vi "MSTAutoSummary.vi"() -> ()   [LabVIEW 2012]
uses:
  <vilib>/Utility/NIReport.llb/NI_report.lvclass
  <vilib>/addons/database/Connection.llb/DB Tools Open Connec (Path).vi
  <vilib>/addons/database/Connection.llb/Conn Execute.vi
  <vilib>/addons/database/Recordset.llb/Rec Fetch Recordset Data (R).vi
  <vilib>/addons/database/Recordset.llb/Rec Destroy - Connection.vi
  <vilib>/Utility/NIReport.llb/Append Text Table to Report (wrap).vi
  <vilib>/addons/database/_DB Variant To Data/Database Variant To Data.xnode
  <vilib>/addons/database/NI_Database_API.lvlib
  <vilib>/Utility/NIReport.llb/Excel/NI_Excel.lvclass
  <vilib>/addons/_office/NI_ReportGenerationToolkit.lvlib
  <vilib>/Utility/SMTP/NI_SMTPEmail.lvlib
panel:
  in  "Report Template":path=path "O:/Monitor/Report/MSTDailyReport.xls"
  in  "Table Control":string[][](table)
  in  "Table Control 2":string[][](table)
  in  "Table Control 3":string[][](table)
  out "error out 4":errorcluster
  out "error out 5":errorcluster
  out "appended array 4":string[](array[string])
  out "recordset data 4":variant[][](array[variant])
  out "error out 3":errorcluster
  out "appended array 3":string[](array[string])
  out "recordset data 3":variant[][](array[variant])
  out "error out":errorcluster
  out "appended array":string[](array[string])
  out "recordset data":variant[][](array[variant])
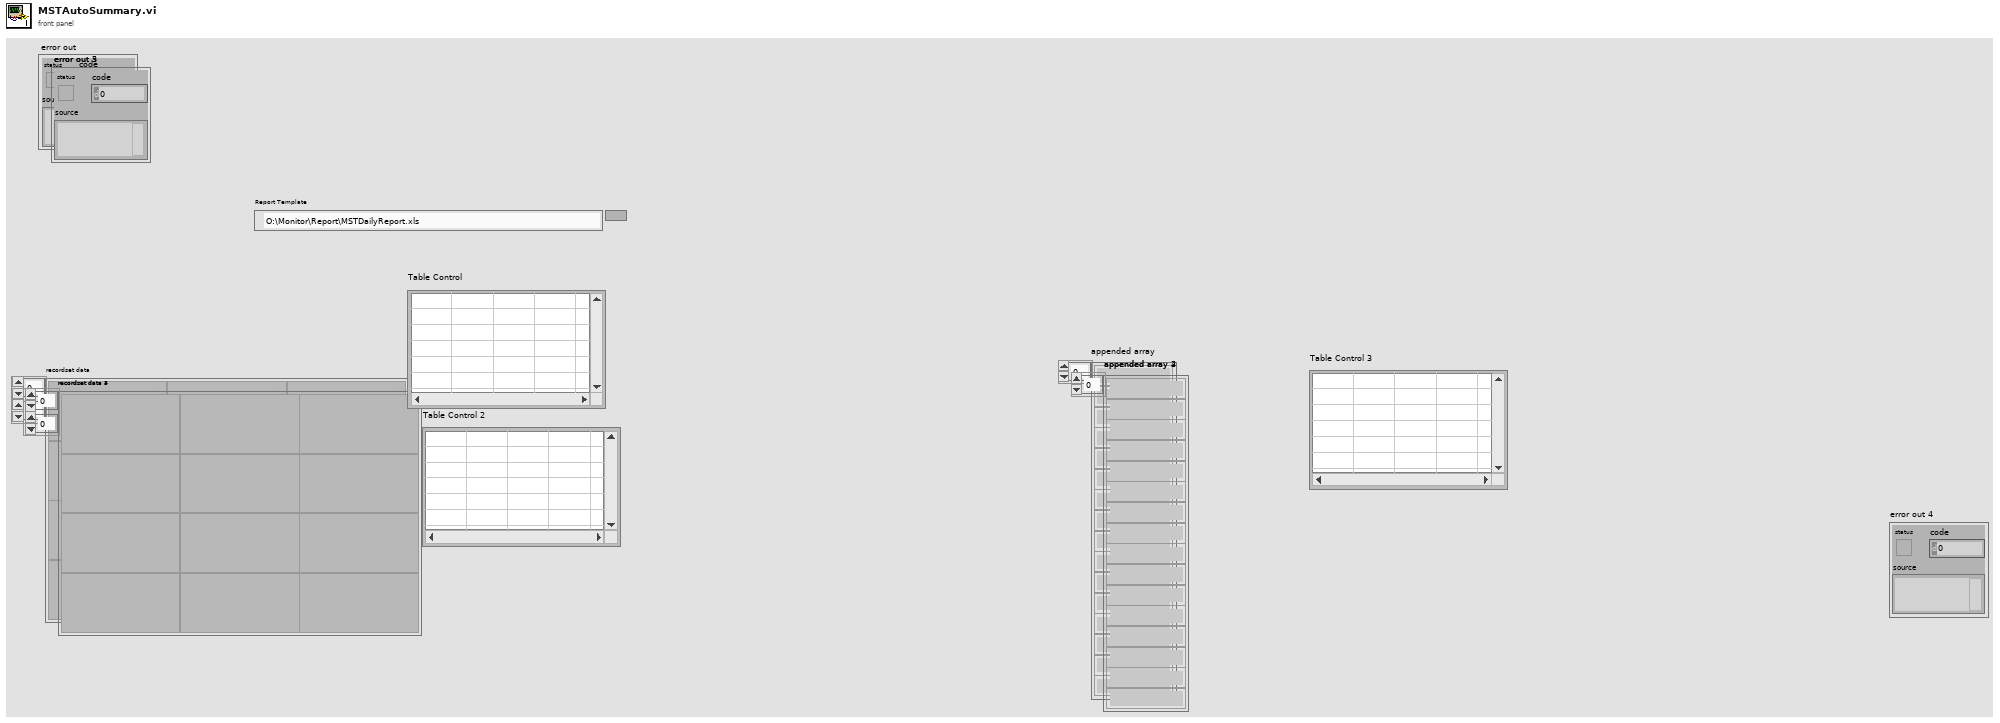
[diagram p1: front panel]
types:
  T1 = typedef "NI_Database_API.lvlib/Conn ObjectReference.ctl" = refnum<k1>
  T2 = typedef "NI_Database_API.lvlib/Rec ObjectReference.ctl" = refnum<k1>
  T3 = enum16{"Standard Report", "HTML", "Word", "Excel"}
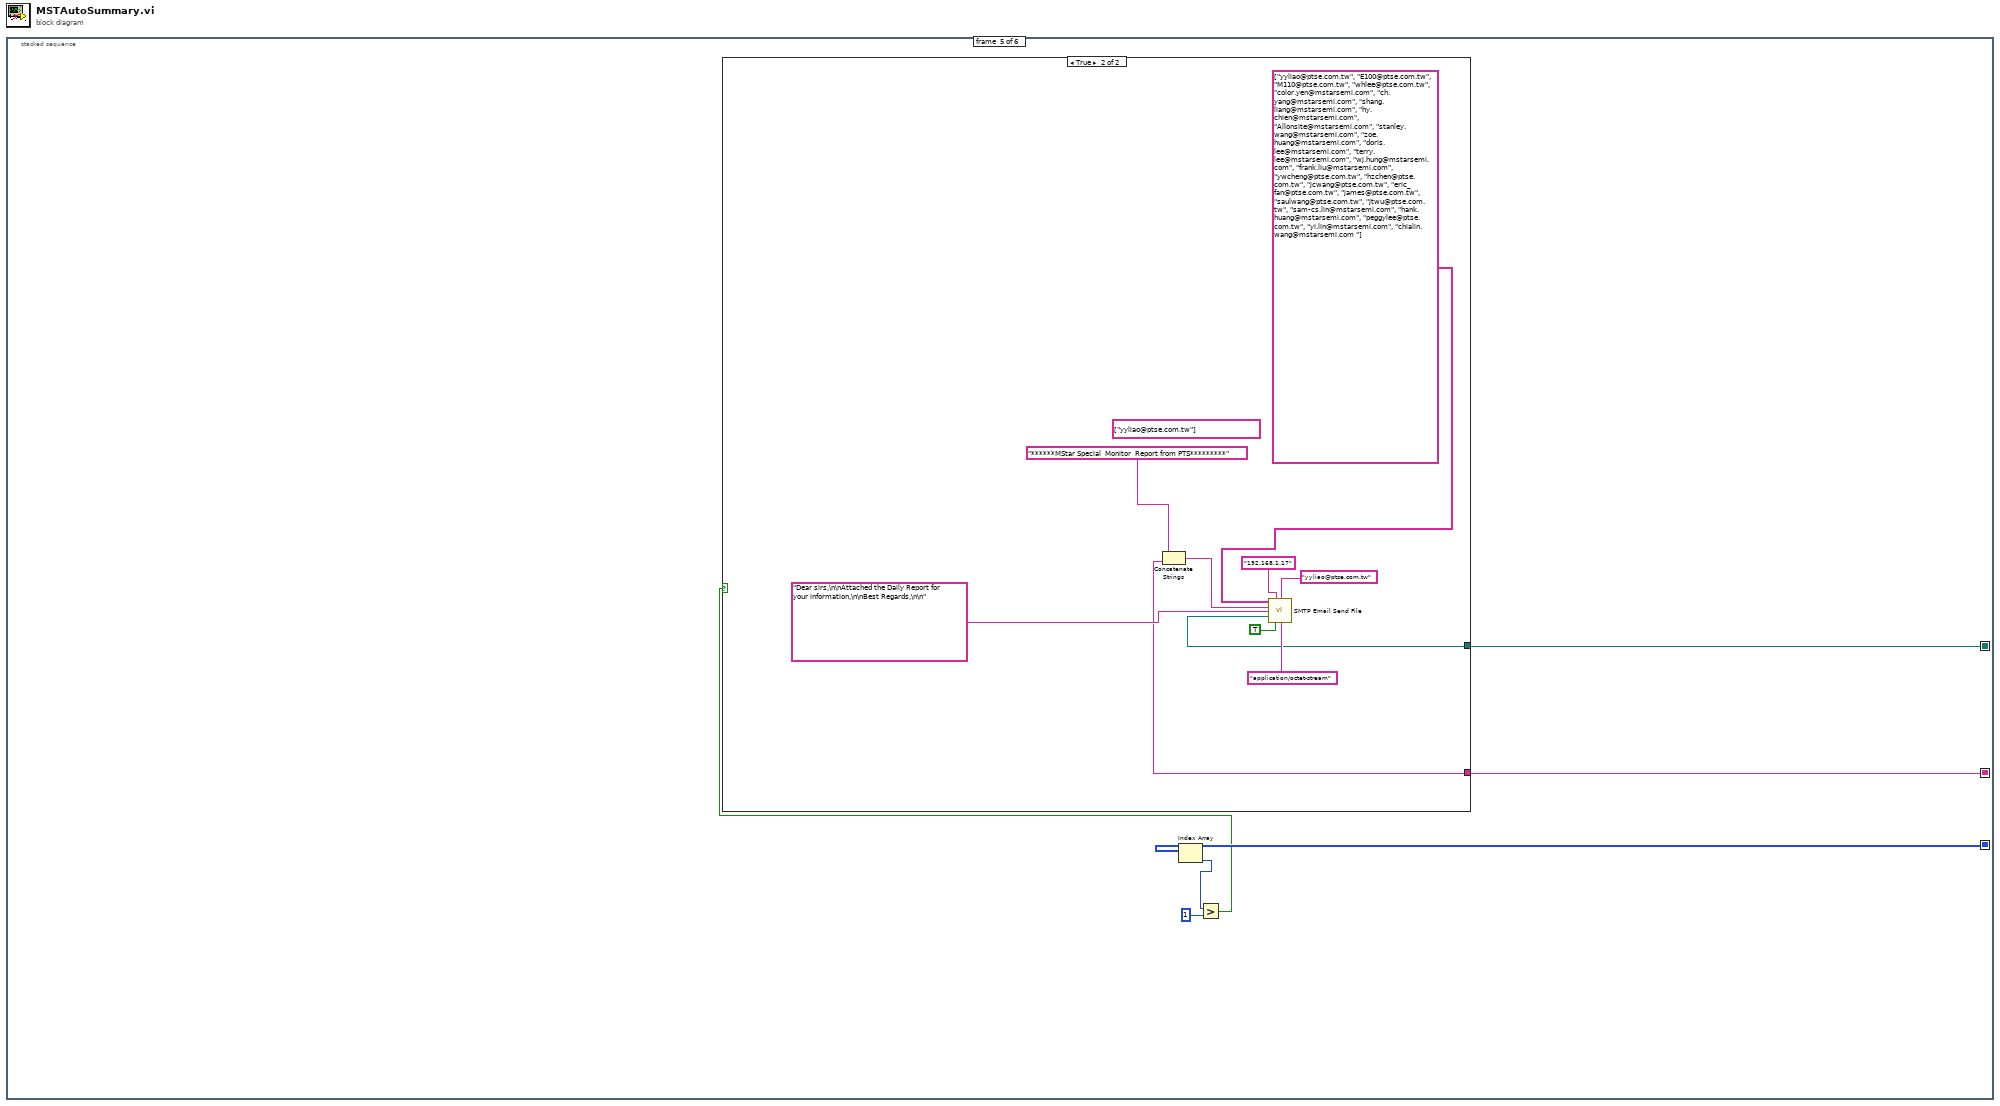
[diagram p0: block diagram]
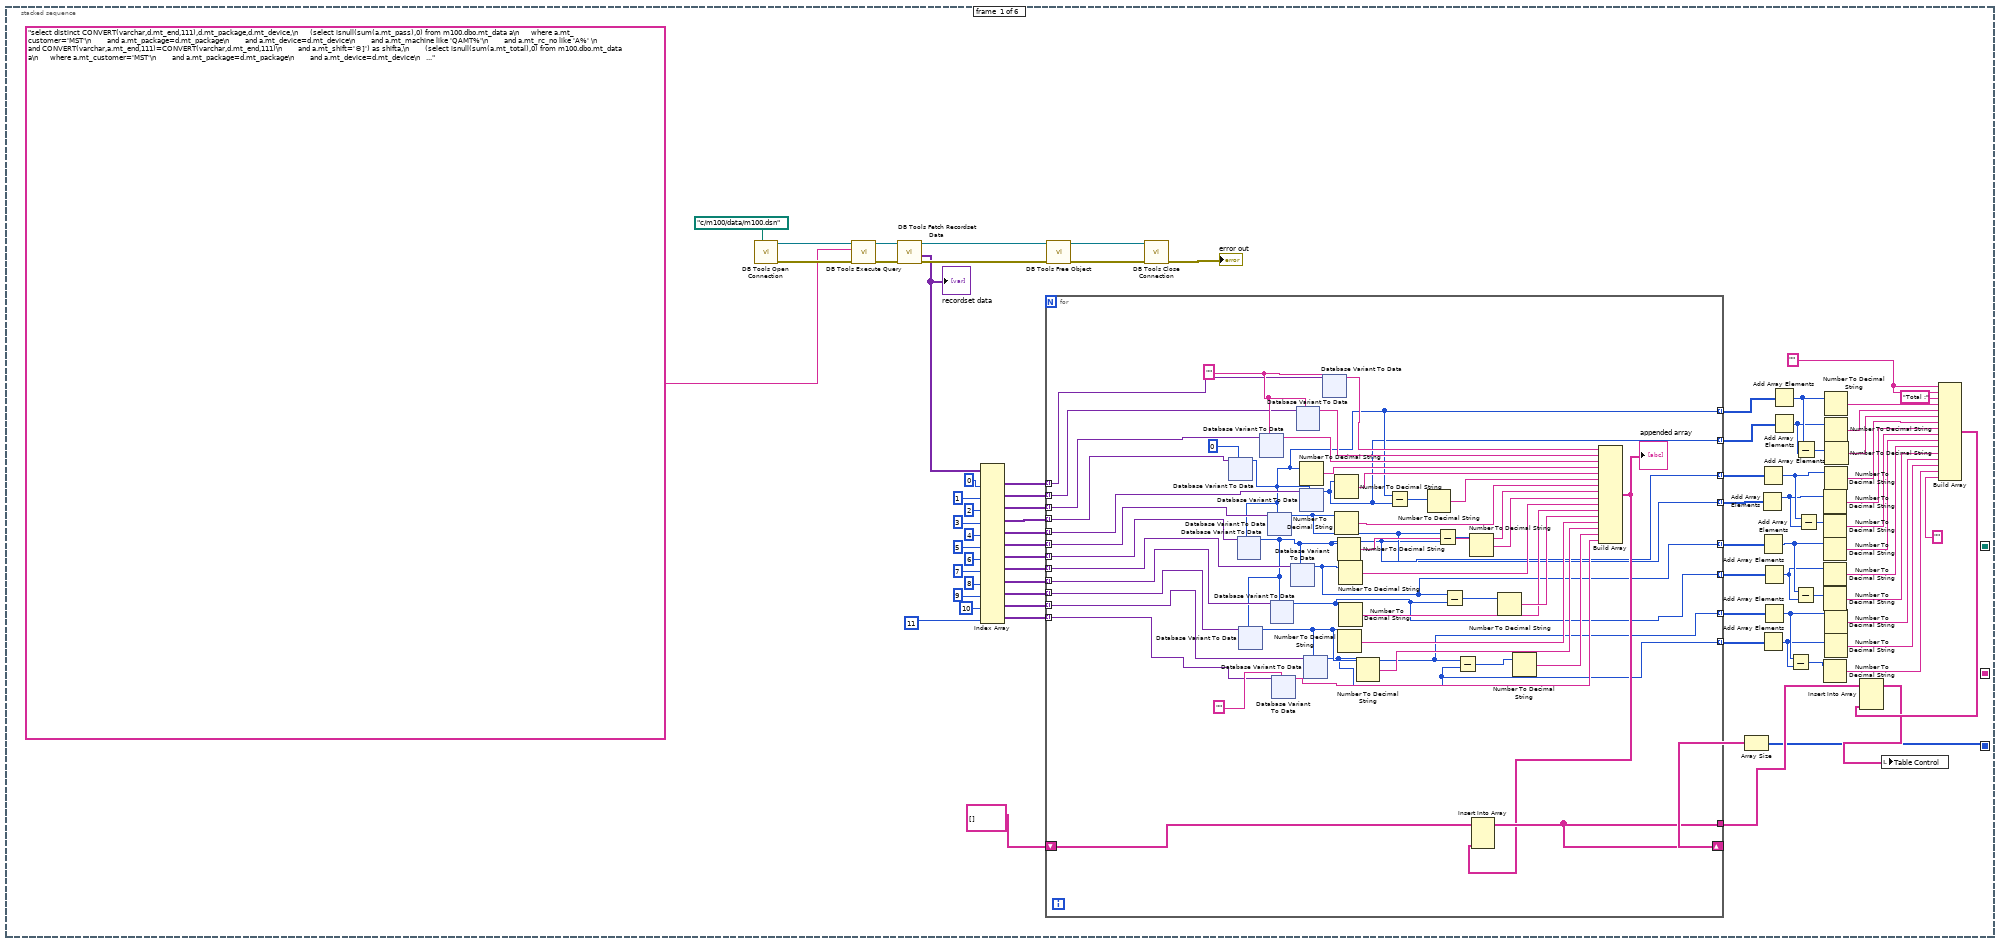
[diagram p2: hidden frame]
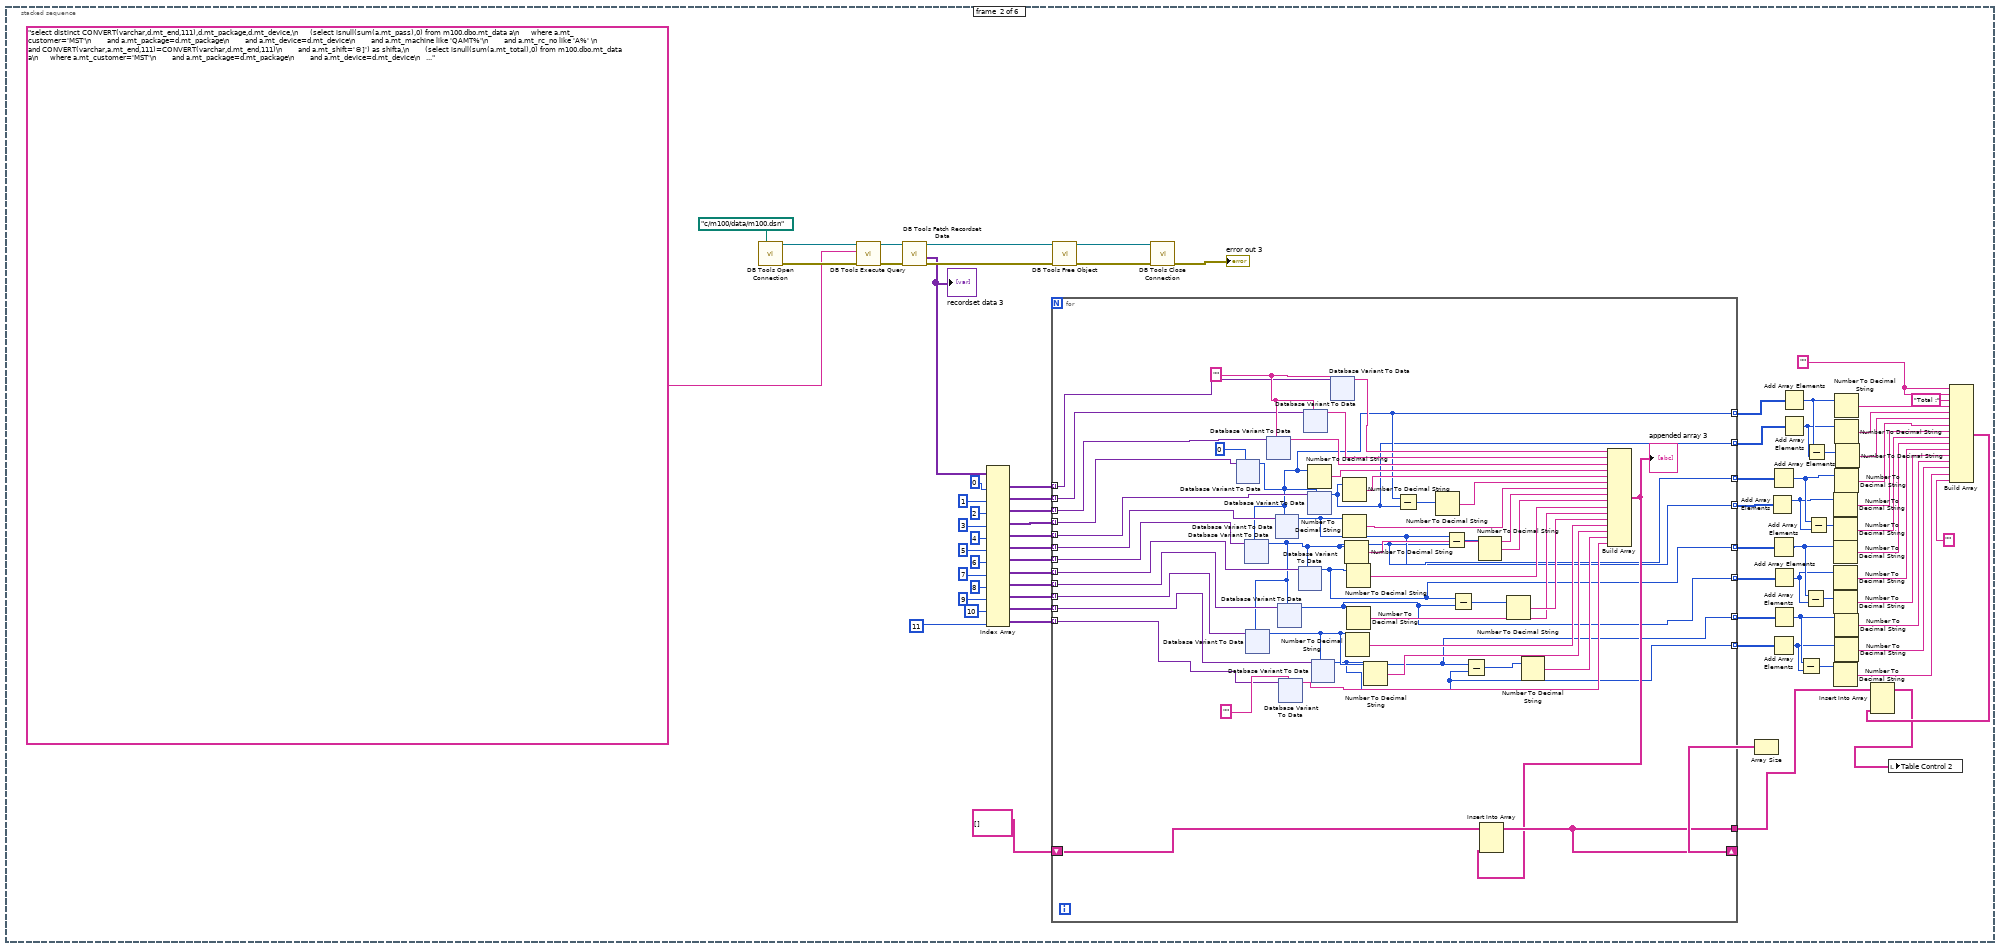
[diagram p3: hidden frame]
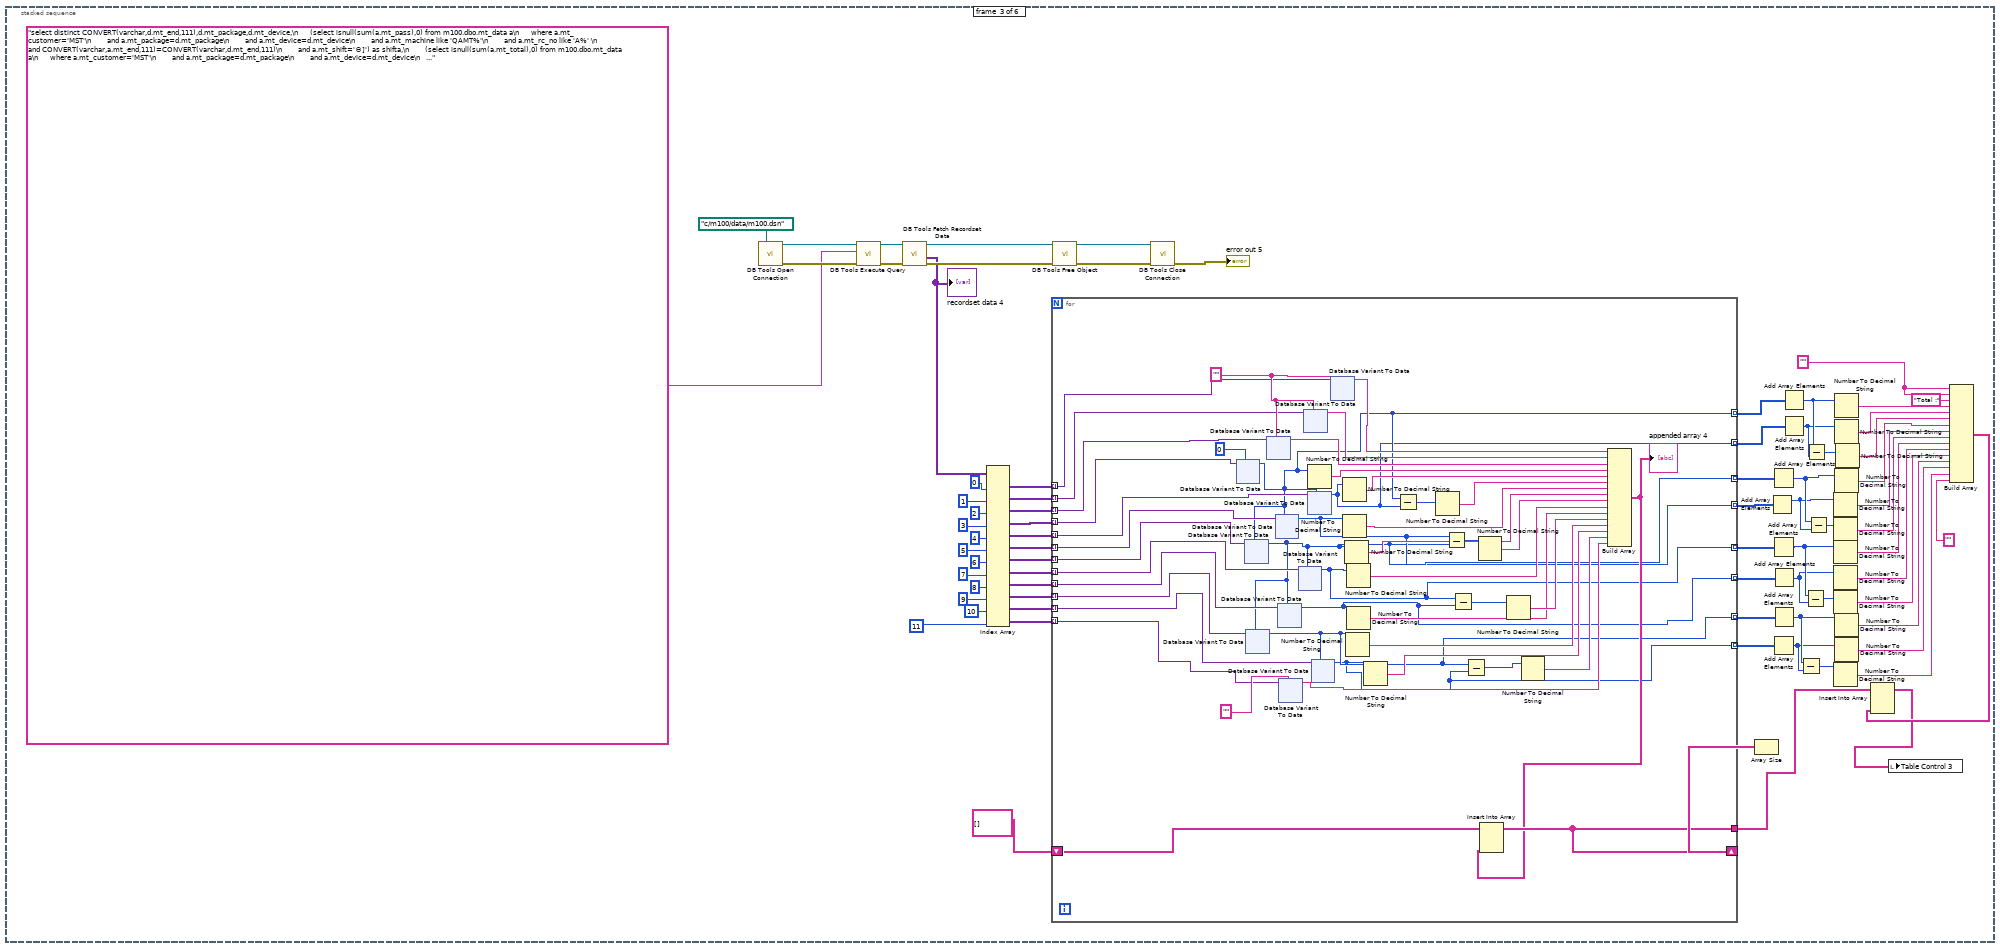
[diagram p4: hidden frame]
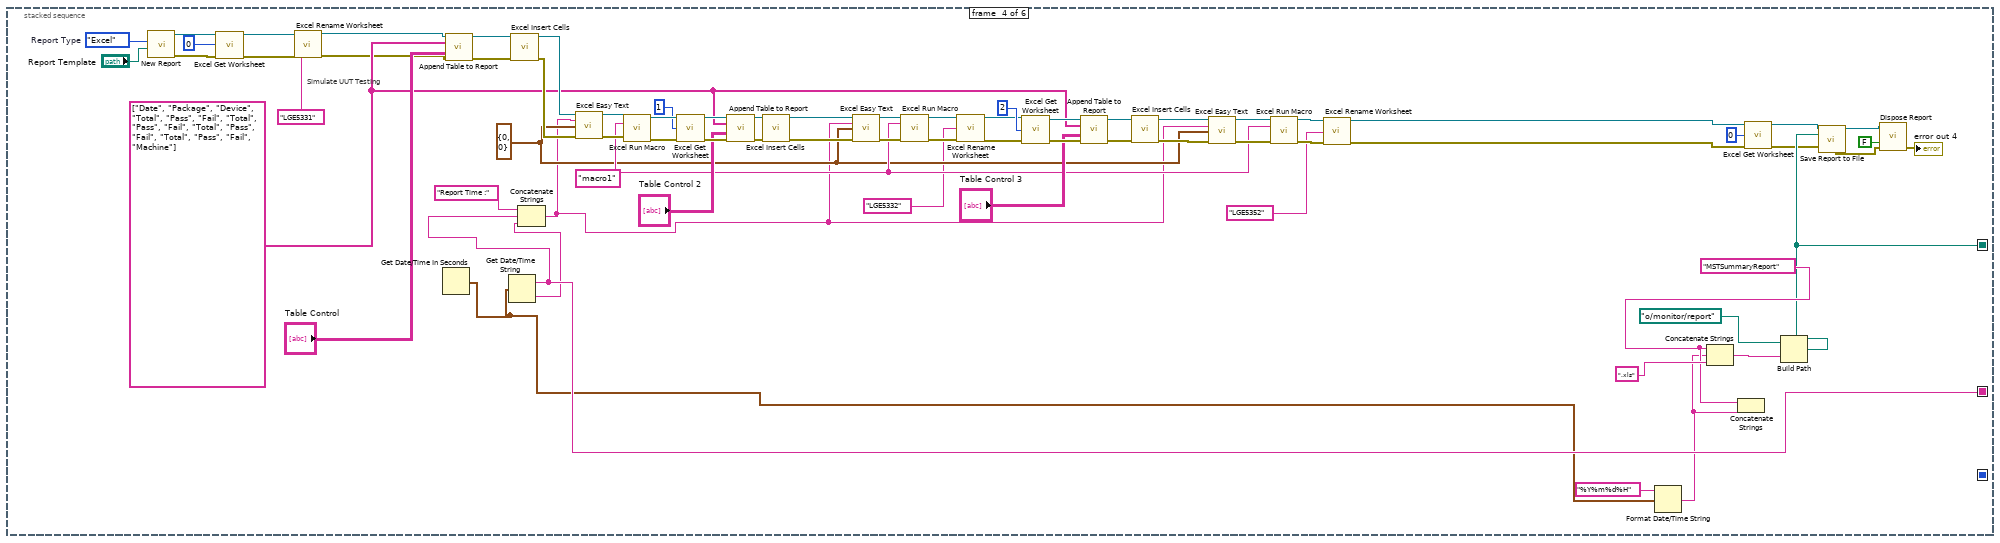
[diagram p5: hidden frame]
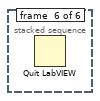
[diagram p7: hidden frame]
diagram:
  n1 = stacked-sequence {
    seq-local: [_ _ _ w1576 _ _] -> [_ _ _ _ w1596 _]
    seq-local: [_ _ _ w1575 _ _] -> [_ _ _ _ w1595 _]
    seq-local: [w1 _ _ _ _ _] -> [_ _ _ _ w1594 _]
    frame #0 {
      w37 = ""
      n2 = call-poly <vilib>:"DB Tools Open Connection.vi"("connection information"=path "c:/m100/data/m100.dsn") -> ("error out"=w72:errorcluster, "connection reference"=w76:T1)  [unwired: 7 in]
      n3 = call-poly <vilib>:"DB Tools Execute Query.vi"("error in (no error)"=w72, "SQL query"="select distinct CONVERT(varchar,d.mt_end,111),d.mt_package,d.mt_device,\n      (select isnull(sum(a.mt_pass),0) from m100.dbo.mt_data a\n      where a.mt_customer='MST'\n        and a.mt_package=d.mt_package\n        and a.mt_device=d.mt_device\n        and a.mt_machine like 'QAMT%'\n        and a.mt_rc_no like 'A%' \n        and CONVERT(varchar,a.mt_end,111)=CONVERT(varchar,d.mt_end,111)\n        and a.mt_shift='©]') as shifta,\n        (select isnull(sum(a.mt_total),0) from m100.dbo.mt_data a\n      where a.mt_customer='MST'\n        and a.mt_package=d.mt_package\n        and a.mt_device=d.mt_device\n        and a.mt_machine like 'QAMT%'\n        and a.mt_rc_no like 'A%' \n        and CONVERT(varchar,a.mt_end,111)=CONVERT(varchar,d.mt_end,111)\n        and a.mt_shift='©]') as shifta1,\n        (select isnull(sum(b.mt_pass),0) from m100.dbo.mt_data b\n      where b.mt_customer='MST'\n        and b.mt_package=d.mt_package\n       and b.mt_device=d.mt_device\n        and b.mt_machine like 'QAMT%'\n        and b.mt_rc_no like 'A%' \n        and CONVERT(varchar,b.mt_end,111)=CONVERT(varchar,d.mt_end,111)\n        and b.mt_shift='¦­') as shiftb,\n        (select isnull(sum(b.mt_total),0) from m100.dbo.mt_data b\n      where b.mt_customer='MST'\n        and b.mt_package=d.mt_package\n        and b.mt_device=d.mt_device\n        and b.mt_machine like 'QAMT%'\n        and b.mt_rc_no like 'A%' \n        and CONVERT(varchar,b.mt_end,111)=CONVERT(varchar,d.mt_end,111)\n        and b.mt_shift='¦­') as shiftb1,\n        (select isnull(sum(c.mt_pass),0) from m100.dbo.mt_data c\n      where c.mt_customer='MST'\n        and c.mt_package=d.mt_package\n        and c.mt_device=d.mt_device\n        and c.mt_machine like 'QAMT%'\n        and c.mt_rc_no like 'A%' \n        and CONVERT(varchar,c.mt_end,111)=CONVERT(varchar,d.mt_end,111)\n        and c.mt_shift='¤¤') as shiftc,\n        (select isnull(sum(c.mt_total),0) from m100.dbo.mt_data c\n      where c.mt_customer='MST'\n        and c.mt_package=d.mt_package\n        and c.mt_device=d.mt_device\n        and c.mt_machine like 'QAMT%'\n        and c.mt_rc_no like 'A%' \n        and CONVERT(varchar,c.mt_end,111)=CONVERT(varchar,d.mt_end,111)\n        and c.mt_shift='¤¤') as shiftc1,\n        SUM(mt_pass),SUM(mt_total),master.dbo.GetEntityNameFromDateToDate('MST',d.mt_package,d.mt_device,CONVERT(varchar,d.mt_end,111),CONVERT(varchar,d.mt_end,111))\n  FROM [m100].[dbo].[mt_data] d\n  WHERE d.mt_customer='MST'\n    and d.mt_machine like 'QAMT%'\n    and d.mt_device='LGE5331'\n    AND CONVERT(varchar,d.mt_end,111) between '2015/08/19' and convert(varchar,getdate(),111)\n    and d.mt_pass > 0 and d.mt_rc_no like 'A%'\n      group by CONVERT(varchar,d.mt_end,111),d.mt_package,d.mt_device", "connection reference"=w76) -> ("error out"=w71:errorcluster, "recordset reference"=w75:T2)  [unwired: 5 in]
      n4 = call-poly <vilib>:"DB Tools Fetch Recordset Data.vi"("error in (no error)"=w71, "recordset reference"=w75) -> ("error out"=w70:errorcluster, "recordset data"=w40:variant[][], "recordset reference out"=w74:T2)  [unwired: 3 in]
      "recordset data" <- w40
      n5 = Index Array(array=w40, index (col) #1=0 ("index (row)"), index (col) #2=1 ("index (col)"), index (col) #3=2 ("disabled index (col)"), index (col) #4=3 ("index (col)"), index (col) #5=4 ("index (col)"), index (col) #6=5 ("index (col)"), index (col) #7=6 ("index (col)"), index (col) #8=7 ("index (col)"), index (col) #9=8 ("index (col)"), index (col) #10=9 ("index (col)"), index (col) #11=10 ("index (col)"), index (col) #12=11 ("index (col)")) -> (element #1=w44:variant[], element #2=w43:variant[], element #3=w57:variant[], element #4=w56:variant[], element #5=w55:variant[], element #6=w54:variant[], element #7=w53:variant[], element #8=w52:variant[], element #9=w51:variant[], element #10=w50:variant[], element #11=w49:variant[], element #12=w48:variant[])  [unwired: 12 in]
      n6 = for {
        tunnel: w57 -> [w96] mode=indexing
        tunnel: w56 -> [w95] mode=indexing
        tunnel: w55 -> [w94] mode=indexing
        tunnel: w54 -> [w93] mode=indexing
        tunnel: w53 -> [w92] mode=indexing
        tunnel: w52 -> [w91] mode=indexing
        tunnel: w51 -> [w90] mode=indexing
        tunnel: w50 -> [w89] mode=indexing
        tunnel: w49 -> [w88] mode=indexing
        tunnel: w48 -> [w87] mode=indexing
        tunnel: [w123] -> w30
        shift-right: [w123] -> w46
        shift-left: string[][] [] ("array") -> [w122]
        tunnel: w44 -> [w98] mode=indexing
        tunnel: w43 -> [w97] mode=indexing
        tunnel: [w85] -> w39 mode=indexing
        tunnel: [w84] -> w38 mode=indexing
        tunnel: [w83] -> w28 mode=indexing
        tunnel: [w82] -> w27 mode=indexing
        tunnel: [w81] -> w18 mode=indexing
        tunnel: [w80] -> w17 mode=indexing
        tunnel: [w79] -> w10 mode=indexing
        tunnel: [w78] -> w9 mode=indexing
        w121 = ""
        n7 = xnode "Database Variant To Data"("database variant"=w95, "type"=0) -> ("data"=w85:i32)  [unwired: 1 in, 1 out]
        n8 = xnode "Database Variant To Data"("database variant"=w92, "type"=w85) -> ("data"=w82:i32)  [unwired: 1 in, 1 out]
        n9 = xnode "Database Variant To Data"("database variant"=w89, "type"=w82) -> ("data"=w79:i32)  [unwired: 1 in, 1 out]
        n10 = xnode "Database Variant To Data"("database variant"=w96, "type"=w121) -> ("data"=w104:string)  [unwired: 1 in, 1 out]
        n11 = xnode "Database Variant To Data"("database variant"=w93, "type"=w85) -> ("data"=w83:i32)  [unwired: 1 in, 1 out]
        n12 = xnode "Database Variant To Data"("database variant"=w90, "type"=w82) -> ("data"=w80:i32)  [unwired: 1 in, 1 out]
        n13 = xnode "Database Variant To Data"("database variant"=w87, "type"="") -> ("data"=w116:string)  [unwired: 1 in, 1 out]
        n14 = xnode "Database Variant To Data"("database variant"=w91, "type"=w82) -> ("data"=w81:i32)  [unwired: 1 in, 1 out]
        n15 = xnode "Database Variant To Data"("database variant"=w97, "type"=w121) -> ("data"=w101:string)  [unwired: 1 in, 1 out]
        n16 = Number To Decimal String(number=w85) -> (decimal integer string=w103:string)  [unwired: 1 in]
        n17 = xnode "Database Variant To Data"("database variant"=w94, "type"=w85) -> ("data"=w84:i32)  [unwired: 1 in, 1 out]
        n18 = xnode "Database Variant To Data"("database variant"=w88, "type"=w79) -> ("data"=w78:i32)  [unwired: 1 in, 1 out]
        n19 = xnode "Database Variant To Data"("database variant"=w98, "type"=w121) -> ("data"=w105:string)  [unwired: 1 in, 1 out]
        n20 = Number To Decimal String(number=w84) -> (decimal integer string=w102:string)  [unwired: 1 in]
        n21 = Number To Decimal String(number=w83) -> (decimal integer string=w119:string)  [unwired: 1 in]
        n22 = Number To Decimal String(number=w82) -> (decimal integer string=w118:string)  [unwired: 1 in]
        n23 = Number To Decimal String(number=w79) -> (decimal integer string=w112:string)  [unwired: 1 in]
        n24 = Number To Decimal String(number=w81) -> (decimal integer string=w108:string)  [unwired: 1 in]
        n25 = Number To Decimal String(number=w80) -> (decimal integer string=w109:string)  [unwired: 1 in]
        n26 = Number To Decimal String(number=w78) -> (decimal integer string=w113:string)  [unwired: 1 in]
        n27 = Subtract(x=w85, y=w84) -> (x-y=w100:i32)
        n28 = Number To Decimal String(number=w100) -> (decimal integer string=w99:string)  [unwired: 1 in]
        n29 = Subtract(x=w83, y=w82) -> (x-y=w107:i32)
        n30 = Subtract(x=w81, y=w80) -> (x-y=w111:i32)
        n31 = Subtract(x=w79, y=w78) -> (x-y=w115:i32)
        n32 = Number To Decimal String(number=w107) -> (decimal integer string=w106:string)  [unwired: 1 in]
        n33 = Number To Decimal String(number=w111) -> (decimal integer string=w110:string)  [unwired: 1 in]
        n34 = Number To Decimal String(number=w115) -> (decimal integer string=w114:string)  [unwired: 1 in]
        n35 = Build Array(w105, w101, w104, w103, w102, w99, w119, w118, w106, w108, w109, w110, w112, w113, w114, w116) -> (w86:string[])
        "appended array" <- w86
        n36 = Insert Into Array(array=w122, new element=w86) -> (w123:string[][])  [unwired: 2 in]
      }
      n37 = call-poly <vilib>:"DB Tools Free Object.vi"("error in (no error)"=w70, "recordset reference"=w74) -> ("error out"=w69:errorcluster, "connection reference"=w73:T1)  [unwired: 8 in]
      n38 = call <vilib>:"DB Tools Close Connection.vi"("error in (no error)"=w69, "connection reference"=w73) -> ("error out"=→"error out":errorcluster)  [unwired: 5 in]
      n39 = Array Size(array=w46) -> (size(s)=w1:i32[])
      n40 = Add Array Elements(numeric array=w27) -> (sum=w21:i32)
      n41 = Add Array Elements(numeric array=w28) -> (sum=w22:i32)
      n42 = Add Array Elements(numeric array=w18) -> (sum=w14:i32)
      n43 = Add Array Elements(numeric array=w9) -> (sum=w7:i32)
      n44 = Add Array Elements(numeric array=w17) -> (sum=w13:i32)
      n45 = Add Array Elements(numeric array=w10) -> (sum=w8:i32)
      n46 = Add Array Elements(numeric array=w39) -> (sum=w34:i32)
      n47 = Add Array Elements(numeric array=w38) -> (sum=w33:i32)
      n48 = Subtract(x=w8, y=w7) -> (x-y=w6:i32)
      n49 = Subtract(x=w14, y=w13) -> (x-y=w11:i32)
      n50 = Subtract(x=w34, y=w33) -> (x-y=w26:i32)
      n51 = Subtract(x=w22, y=w21) -> (x-y=w19:i32)
      n52 = Number To Decimal String(number=w21) -> (decimal integer string=w23:string)  [unwired: 1 in]
      n53 = Number To Decimal String(number=w19) -> (decimal integer string=w20:string)  [unwired: 1 in]
      n54 = Number To Decimal String(number=w14) -> (decimal integer string=w16:string)  [unwired: 1 in]
      n55 = Number To Decimal String(number=w13) -> (decimal integer string=w15:string)  [unwired: 1 in]
      n56 = Number To Decimal String(number=w11) -> (decimal integer string=w12:string)  [unwired: 1 in]
      n57 = Number To Decimal String(number=w6) -> (decimal integer string=w3:string)  [unwired: 1 in]
      n58 = Number To Decimal String(number=w34) -> (decimal integer string=w36:string)  [unwired: 1 in]
      n59 = Number To Decimal String(number=w33) -> (decimal integer string=w35:string)  [unwired: 1 in]
      n60 = Number To Decimal String(number=w22) -> (decimal integer string=w25:string)  [unwired: 1 in]
      n61 = Number To Decimal String(number=w8) -> (decimal integer string=w5:string)  [unwired: 1 in]
      n62 = Number To Decimal String(number=w7) -> (decimal integer string=w4:string)  [unwired: 1 in]
      n63 = Number To Decimal String(number=w26) -> (decimal integer string=w32:string)  [unwired: 1 in]
      n64 = Build Array(w37, w37, "Total :" ("element"), w36, w35, w32, w25, w23, w20, w16, w15, w12, w5, w4, w3, "") -> (w31:string[])
      n65 = Insert Into Array(array=w30, new element=w31) -> (w29:string[][])  [unwired: 2 in]
      n66 = local write "Table Control"(w29) -> ()
    }
    frame #1 {
      w543 = ""
      n67 = call-poly <vilib>:"DB Tools Open Connection.vi"("connection information"=path "c:/m100/data/m100.dsn") -> ("error out"=w578:errorcluster, "connection reference"=w582:T1)  [unwired: 7 in]
      n68 = call-poly <vilib>:"DB Tools Execute Query.vi"("error in (no error)"=w578, "SQL query"="select distinct CONVERT(varchar,d.mt_end,111),d.mt_package,d.mt_device,\n      (select isnull(sum(a.mt_pass),0) from m100.dbo.mt_data a\n      where a.mt_customer='MST'\n        and a.mt_package=d.mt_package\n        and a.mt_device=d.mt_device\n        and a.mt_machine like 'QAMT%'\n        and a.mt_rc_no like 'A%' \n        and CONVERT(varchar,a.mt_end,111)=CONVERT(varchar,d.mt_end,111)\n        and a.mt_shift='©]') as shifta,\n        (select isnull(sum(a.mt_total),0) from m100.dbo.mt_data a\n      where a.mt_customer='MST'\n        and a.mt_package=d.mt_package\n        and a.mt_device=d.mt_device\n        and a.mt_machine like 'QAMT%'\n        and a.mt_rc_no like 'A%' \n        and CONVERT(varchar,a.mt_end,111)=CONVERT(varchar,d.mt_end,111)\n        and a.mt_shift='©]') as shifta1,\n        (select isnull(sum(b.mt_pass),0) from m100.dbo.mt_data b\n      where b.mt_customer='MST'\n        and b.mt_package=d.mt_package\n       and b.mt_device=d.mt_device\n        and b.mt_machine like 'QAMT%'\n        and b.mt_rc_no like 'A%' \n        and CONVERT(varchar,b.mt_end,111)=CONVERT(varchar,d.mt_end,111)\n        and b.mt_shift='¦­') as shiftb,\n        (select isnull(sum(b.mt_total),0) from m100.dbo.mt_data b\n      where b.mt_customer='MST'\n        and b.mt_package=d.mt_package\n        and b.mt_device=d.mt_device\n        and b.mt_machine like 'QAMT%'\n        and b.mt_rc_no like 'A%' \n        and CONVERT(varchar,b.mt_end,111)=CONVERT(varchar,d.mt_end,111)\n        and b.mt_shift='¦­') as shiftb1,\n        (select isnull(sum(c.mt_pass),0) from m100.dbo.mt_data c\n      where c.mt_customer='MST'\n        and c.mt_package=d.mt_package\n        and c.mt_device=d.mt_device\n        and c.mt_machine like 'QAMT%'\n        and c.mt_rc_no like 'A%' \n        and CONVERT(varchar,c.mt_end,111)=CONVERT(varchar,d.mt_end,111)\n        and c.mt_shift='¤¤') as shiftc,\n        (select isnull(sum(c.mt_total),0) from m100.dbo.mt_data c\n      where c.mt_customer='MST'\n        and c.mt_package=d.mt_package\n        and c.mt_device=d.mt_device\n        and c.mt_machine like 'QAMT%'\n        and c.mt_rc_no like 'A%' \n        and CONVERT(varchar,c.mt_end,111)=CONVERT(varchar,d.mt_end,111)\n        and c.mt_shift='¤¤') as shiftc1,\n        SUM(mt_pass),SUM(mt_total),master.dbo.GetEntityNameFromDateToDate('MST',d.mt_package,d.mt_device,CONVERT(varchar,d.mt_end,111),CONVERT(varchar,d.mt_end,111))\n  FROM [m100].[dbo].[mt_data] d\n  WHERE d.mt_customer='MST'\n    and d.mt_machine like 'QAMT%'\n    and d.mt_device='LGE5332'\n    AND CONVERT(varchar,d.mt_end,111) between '2015/08/19' and convert(varchar,getdate(),111)\n    and d.mt_pass > 0 and d.mt_rc_no like 'A%'\n      group by CONVERT(varchar,d.mt_end,111),d.mt_package,d.mt_device", "connection reference"=w582) -> ("error out"=w577:errorcluster, "recordset reference"=w581:T2)  [unwired: 5 in]
      n69 = call-poly <vilib>:"DB Tools Fetch Recordset Data.vi"("error in (no error)"=w577, "recordset reference"=w581) -> ("error out"=w576:errorcluster, "recordset data"=w546:variant[][], "recordset reference out"=w580:T2)  [unwired: 3 in]
      "recordset data 3" <- w546
      n70 = Index Array(array=w546, index (col) #1=0 ("index (row)"), index (col) #2=1 ("index (col)"), index (col) #3=2 ("disabled index (col)"), index (col) #4=3 ("index (col)"), index (col) #5=4 ("index (col)"), index (col) #6=5 ("index (col)"), index (col) #7=6 ("index (col)"), index (col) #8=7 ("index (col)"), index (col) #9=8 ("index (col)"), index (col) #10=9 ("index (col)"), index (col) #11=10 ("index (col)"), index (col) #12=11 ("index (col)")) -> (element #1=w550:variant[], element #2=w549:variant[], element #3=w563:variant[], element #4=w562:variant[], element #5=w561:variant[], element #6=w560:variant[], element #7=w559:variant[], element #8=w558:variant[], element #9=w557:variant[], element #10=w556:variant[], element #11=w555:variant[], element #12=w554:variant[])  [unwired: 12 in]
      n71 = for {
        tunnel: w563 -> [w602] mode=indexing
        tunnel: w562 -> [w601] mode=indexing
        tunnel: w561 -> [w600] mode=indexing
        tunnel: w560 -> [w599] mode=indexing
        tunnel: w559 -> [w598] mode=indexing
        tunnel: w558 -> [w597] mode=indexing
        tunnel: w557 -> [w596] mode=indexing
        tunnel: w556 -> [w595] mode=indexing
        tunnel: w555 -> [w594] mode=indexing
        tunnel: w554 -> [w593] mode=indexing
        tunnel: [w629] -> w536
        shift-right: [w629] -> w552
        shift-left: string[][] [] ("array") -> [w628]
        tunnel: w550 -> [w604] mode=indexing
        tunnel: w549 -> [w603] mode=indexing
        tunnel: [w591] -> w545 mode=indexing
        tunnel: [w590] -> w544 mode=indexing
        tunnel: [w589] -> w534 mode=indexing
        tunnel: [w588] -> w533 mode=indexing
        tunnel: [w587] -> w524 mode=indexing
        tunnel: [w586] -> w523 mode=indexing
        tunnel: [w585] -> w516 mode=indexing
        tunnel: [w584] -> w515 mode=indexing
        w627 = ""
        n72 = xnode "Database Variant To Data"("database variant"=w601, "type"=0) -> ("data"=w591:i32)  [unwired: 1 in, 1 out]
        n73 = xnode "Database Variant To Data"("database variant"=w598, "type"=w591) -> ("data"=w588:i32)  [unwired: 1 in, 1 out]
        n74 = xnode "Database Variant To Data"("database variant"=w595, "type"=w588) -> ("data"=w585:i32)  [unwired: 1 in, 1 out]
        n75 = xnode "Database Variant To Data"("database variant"=w602, "type"=w627) -> ("data"=w610:string)  [unwired: 1 in, 1 out]
        n76 = xnode "Database Variant To Data"("database variant"=w599, "type"=w591) -> ("data"=w589:i32)  [unwired: 1 in, 1 out]
        n77 = xnode "Database Variant To Data"("database variant"=w596, "type"=w588) -> ("data"=w586:i32)  [unwired: 1 in, 1 out]
        n78 = xnode "Database Variant To Data"("database variant"=w593, "type"="") -> ("data"=w622:string)  [unwired: 1 in, 1 out]
        n79 = xnode "Database Variant To Data"("database variant"=w597, "type"=w588) -> ("data"=w587:i32)  [unwired: 1 in, 1 out]
        n80 = xnode "Database Variant To Data"("database variant"=w603, "type"=w627) -> ("data"=w607:string)  [unwired: 1 in, 1 out]
        n81 = Number To Decimal String(number=w591) -> (decimal integer string=w609:string)  [unwired: 1 in]
        n82 = xnode "Database Variant To Data"("database variant"=w600, "type"=w591) -> ("data"=w590:i32)  [unwired: 1 in, 1 out]
        n83 = xnode "Database Variant To Data"("database variant"=w594, "type"=w585) -> ("data"=w584:i32)  [unwired: 1 in, 1 out]
        n84 = xnode "Database Variant To Data"("database variant"=w604, "type"=w627) -> ("data"=w611:string)  [unwired: 1 in, 1 out]
        n85 = Number To Decimal String(number=w590) -> (decimal integer string=w608:string)  [unwired: 1 in]
        n86 = Number To Decimal String(number=w589) -> (decimal integer string=w625:string)  [unwired: 1 in]
        n87 = Number To Decimal String(number=w588) -> (decimal integer string=w624:string)  [unwired: 1 in]
        n88 = Number To Decimal String(number=w585) -> (decimal integer string=w618:string)  [unwired: 1 in]
        n89 = Number To Decimal String(number=w587) -> (decimal integer string=w614:string)  [unwired: 1 in]
        n90 = Number To Decimal String(number=w586) -> (decimal integer string=w615:string)  [unwired: 1 in]
        n91 = Number To Decimal String(number=w584) -> (decimal integer string=w619:string)  [unwired: 1 in]
        n92 = Subtract(x=w591, y=w590) -> (x-y=w606:i32)
        n93 = Number To Decimal String(number=w606) -> (decimal integer string=w605:string)  [unwired: 1 in]
        n94 = Subtract(x=w589, y=w588) -> (x-y=w613:i32)
        n95 = Subtract(x=w587, y=w586) -> (x-y=w617:i32)
        n96 = Subtract(x=w585, y=w584) -> (x-y=w621:i32)
        n97 = Number To Decimal String(number=w613) -> (decimal integer string=w612:string)  [unwired: 1 in]
        n98 = Number To Decimal String(number=w617) -> (decimal integer string=w616:string)  [unwired: 1 in]
        n99 = Number To Decimal String(number=w621) -> (decimal integer string=w620:string)  [unwired: 1 in]
        n100 = Build Array(w611, w607, w610, w609, w608, w605, w625, w624, w612, w614, w615, w616, w618, w619, w620, w622) -> (w592:string[])
        "appended array 3" <- w592
        n101 = Insert Into Array(array=w628, new element=w592) -> (w629:string[][])  [unwired: 2 in]
      }
      n102 = call-poly <vilib>:"DB Tools Free Object.vi"("error in (no error)"=w576, "recordset reference"=w580) -> ("error out"=w575:errorcluster, "connection reference"=w579:T1)  [unwired: 8 in]
      n103 = call <vilib>:"DB Tools Close Connection.vi"("error in (no error)"=w575, "connection reference"=w579) -> ("error out"=→"error out 3":errorcluster)  [unwired: 5 in]
      n104 = Array Size(array=w552) -> ()  [unwired: 1 out]
      n105 = Add Array Elements(numeric array=w533) -> (sum=w527:i32)
      n106 = Add Array Elements(numeric array=w534) -> (sum=w528:i32)
      n107 = Add Array Elements(numeric array=w524) -> (sum=w520:i32)
      n108 = Add Array Elements(numeric array=w515) -> (sum=w513:i32)
      n109 = Add Array Elements(numeric array=w523) -> (sum=w519:i32)
      n110 = Add Array Elements(numeric array=w516) -> (sum=w514:i32)
      n111 = Add Array Elements(numeric array=w545) -> (sum=w540:i32)
      n112 = Add Array Elements(numeric array=w544) -> (sum=w539:i32)
      n113 = Subtract(x=w514, y=w513) -> (x-y=w512:i32)
      n114 = Subtract(x=w520, y=w519) -> (x-y=w517:i32)
      n115 = Subtract(x=w540, y=w539) -> (x-y=w532:i32)
      n116 = Subtract(x=w528, y=w527) -> (x-y=w525:i32)
      n117 = Number To Decimal String(number=w527) -> (decimal integer string=w529:string)  [unwired: 1 in]
      n118 = Number To Decimal String(number=w525) -> (decimal integer string=w526:string)  [unwired: 1 in]
      n119 = Number To Decimal String(number=w520) -> (decimal integer string=w522:string)  [unwired: 1 in]
      n120 = Number To Decimal String(number=w519) -> (decimal integer string=w521:string)  [unwired: 1 in]
      n121 = Number To Decimal String(number=w517) -> (decimal integer string=w518:string)  [unwired: 1 in]
      n122 = Number To Decimal String(number=w512) -> (decimal integer string=w509:string)  [unwired: 1 in]
      n123 = Number To Decimal String(number=w540) -> (decimal integer string=w542:string)  [unwired: 1 in]
      n124 = Number To Decimal String(number=w539) -> (decimal integer string=w541:string)  [unwired: 1 in]
      n125 = Number To Decimal String(number=w528) -> (decimal integer string=w531:string)  [unwired: 1 in]
      n126 = Number To Decimal String(number=w514) -> (decimal integer string=w511:string)  [unwired: 1 in]
      n127 = Number To Decimal String(number=w513) -> (decimal integer string=w510:string)  [unwired: 1 in]
      n128 = Number To Decimal String(number=w532) -> (decimal integer string=w538:string)  [unwired: 1 in]
      n129 = Build Array(w543, w543, "Total :" ("element"), w542, w541, w538, w531, w529, w526, w522, w521, w518, w511, w510, w509, "") -> (w537:string[])
      n130 = Insert Into Array(array=w536, new element=w537) -> (w535:string[][])  [unwired: 2 in]
      n131 = local write "Table Control 2"(w535) -> ()
    }
    frame #2 {
      w1049 = ""
      n132 = call-poly <vilib>:"DB Tools Open Connection.vi"("connection information"=path "c:/m100/data/m100.dsn") -> ("error out"=w1084:errorcluster, "connection reference"=w1088:T1)  [unwired: 7 in]
      n133 = call-poly <vilib>:"DB Tools Execute Query.vi"("error in (no error)"=w1084, "SQL query"="select distinct CONVERT(varchar,d.mt_end,111),d.mt_package,d.mt_device,\n      (select isnull(sum(a.mt_pass),0) from m100.dbo.mt_data a\n      where a.mt_customer='MST'\n        and a.mt_package=d.mt_package\n        and a.mt_device=d.mt_device\n        and a.mt_machine like 'QAMT%'\n        and a.mt_rc_no like 'A%' \n        and CONVERT(varchar,a.mt_end,111)=CONVERT(varchar,d.mt_end,111)\n        and a.mt_shift='©]') as shifta,\n        (select isnull(sum(a.mt_total),0) from m100.dbo.mt_data a\n      where a.mt_customer='MST'\n        and a.mt_package=d.mt_package\n        and a.mt_device=d.mt_device\n        and a.mt_machine like 'QAMT%'\n        and a.mt_rc_no like 'A%' \n        and CONVERT(varchar,a.mt_end,111)=CONVERT(varchar,d.mt_end,111)\n        and a.mt_shift='©]') as shifta1,\n        (select isnull(sum(b.mt_pass),0) from m100.dbo.mt_data b\n      where b.mt_customer='MST'\n        and b.mt_package=d.mt_package\n       and b.mt_device=d.mt_device\n        and b.mt_machine like 'QAMT%'\n        and b.mt_rc_no like 'A%' \n        and CONVERT(varchar,b.mt_end,111)=CONVERT(varchar,d.mt_end,111)\n        and b.mt_shift='¦­') as shiftb,\n        (select isnull(sum(b.mt_total),0) from m100.dbo.mt_data b\n      where b.mt_customer='MST'\n        and b.mt_package=d.mt_package\n        and b.mt_device=d.mt_device\n        and b.mt_machine like 'QAMT%'\n        and b.mt_rc_no like 'A%' \n        and CONVERT(varchar,b.mt_end,111)=CONVERT(varchar,d.mt_end,111)\n        and b.mt_shift='¦­') as shiftb1,\n        (select isnull(sum(c.mt_pass),0) from m100.dbo.mt_data c\n      where c.mt_customer='MST'\n        and c.mt_package=d.mt_package\n        and c.mt_device=d.mt_device\n        and c.mt_machine like 'QAMT%'\n        and c.mt_rc_no like 'A%' \n        and CONVERT(varchar,c.mt_end,111)=CONVERT(varchar,d.mt_end,111)\n        and c.mt_shift='¤¤') as shiftc,\n        (select isnull(sum(c.mt_total),0) from m100.dbo.mt_data c\n      where c.mt_customer='MST'\n        and c.mt_package=d.mt_package\n        and c.mt_device=d.mt_device\n        and c.mt_machine like 'QAMT%'\n        and c.mt_rc_no like 'A%' \n        and CONVERT(varchar,c.mt_end,111)=CONVERT(varchar,d.mt_end,111)\n        and c.mt_shift='¤¤') as shiftc1,\n        SUM(mt_pass),SUM(mt_total),master.dbo.GetEntityNameFromDateToDate('MST',d.mt_package,d.mt_device,CONVERT(varchar,d.mt_end,111),CONVERT(varchar,d.mt_end,111))\n  FROM [m100].[dbo].[mt_data] d\n  WHERE d.mt_customer='MST'\n    and d.mt_machine like 'QAMT%'\n    and d.mt_device='LGE5352 '\n    AND CONVERT(varchar,d.mt_end,111) between '2015/08/19' and convert(varchar,getdate(),111)\n    and d.mt_pass > 0 and d.mt_rc_no like 'A%'\n      group by CONVERT(varchar,d.mt_end,111),d.mt_package,d.mt_device", "connection reference"=w1088) -> ("error out"=w1083:errorcluster, "recordset reference"=w1087:T2)  [unwired: 5 in]
      n134 = call-poly <vilib>:"DB Tools Fetch Recordset Data.vi"("error in (no error)"=w1083, "recordset reference"=w1087) -> ("error out"=w1082:errorcluster, "recordset data"=w1052:variant[][], "recordset reference out"=w1086:T2)  [unwired: 3 in]
      "recordset data 4" <- w1052
      n135 = Index Array(array=w1052, index (col) #1=0 ("index (row)"), index (col) #2=1 ("index (col)"), index (col) #3=2 ("disabled index (col)"), index (col) #4=3 ("index (col)"), index (col) #5=4 ("index (col)"), index (col) #6=5 ("index (col)"), index (col) #7=6 ("index (col)"), index (col) #8=7 ("index (col)"), index (col) #9=8 ("index (col)"), index (col) #10=9 ("index (col)"), index (col) #11=10 ("index (col)"), index (col) #12=11 ("index (col)")) -> (element #1=w1056:variant[], element #2=w1055:variant[], element #3=w1069:variant[], element #4=w1068:variant[], element #5=w1067:variant[], element #6=w1066:variant[], element #7=w1065:variant[], element #8=w1064:variant[], element #9=w1063:variant[], element #10=w1062:variant[], element #11=w1061:variant[], element #12=w1060:variant[])  [unwired: 12 in]
      n136 = for {
        tunnel: w1069 -> [w1108] mode=indexing
        tunnel: w1068 -> [w1107] mode=indexing
        tunnel: w1067 -> [w1106] mode=indexing
        tunnel: w1066 -> [w1105] mode=indexing
        tunnel: w1065 -> [w1104] mode=indexing
        tunnel: w1064 -> [w1103] mode=indexing
        tunnel: w1063 -> [w1102] mode=indexing
        tunnel: w1062 -> [w1101] mode=indexing
        tunnel: w1061 -> [w1100] mode=indexing
        tunnel: w1060 -> [w1099] mode=indexing
        tunnel: [w1135] -> w1042
        shift-right: [w1135] -> w1058
        shift-left: string[][] [] ("array") -> [w1134]
        tunnel: w1056 -> [w1110] mode=indexing
        tunnel: w1055 -> [w1109] mode=indexing
        tunnel: [w1097] -> w1051 mode=indexing
        tunnel: [w1096] -> w1050 mode=indexing
        tunnel: [w1095] -> w1040 mode=indexing
        tunnel: [w1094] -> w1039 mode=indexing
        tunnel: [w1093] -> w1030 mode=indexing
        tunnel: [w1092] -> w1029 mode=indexing
        tunnel: [w1091] -> w1022 mode=indexing
        tunnel: [w1090] -> w1021 mode=indexing
        w1133 = ""
        n137 = xnode "Database Variant To Data"("database variant"=w1107, "type"=0) -> ("data"=w1097:i32)  [unwired: 1 in, 1 out]
        n138 = xnode "Database Variant To Data"("database variant"=w1104, "type"=w1097) -> ("data"=w1094:i32)  [unwired: 1 in, 1 out]
        n139 = xnode "Database Variant To Data"("database variant"=w1101, "type"=w1094) -> ("data"=w1091:i32)  [unwired: 1 in, 1 out]
        n140 = xnode "Database Variant To Data"("database variant"=w1108, "type"=w1133) -> ("data"=w1116:string)  [unwired: 1 in, 1 out]
        n141 = xnode "Database Variant To Data"("database variant"=w1105, "type"=w1097) -> ("data"=w1095:i32)  [unwired: 1 in, 1 out]
        n142 = xnode "Database Variant To Data"("database variant"=w1102, "type"=w1094) -> ("data"=w1092:i32)  [unwired: 1 in, 1 out]
        n143 = xnode "Database Variant To Data"("database variant"=w1099, "type"="") -> ("data"=w1128:string)  [unwired: 1 in, 1 out]
        n144 = xnode "Database Variant To Data"("database variant"=w1103, "type"=w1094) -> ("data"=w1093:i32)  [unwired: 1 in, 1 out]
        n145 = xnode "Database Variant To Data"("database variant"=w1109, "type"=w1133) -> ("data"=w1113:string)  [unwired: 1 in, 1 out]
        n146 = Number To Decimal String(number=w1097) -> (decimal integer string=w1115:string)  [unwired: 1 in]
        n147 = xnode "Database Variant To Data"("database variant"=w1106, "type"=w1097) -> ("data"=w1096:i32)  [unwired: 1 in, 1 out]
        n148 = xnode "Database Variant To Data"("database variant"=w1100, "type"=w1091) -> ("data"=w1090:i32)  [unwired: 1 in, 1 out]
        n149 = xnode "Database Variant To Data"("database variant"=w1110, "type"=w1133) -> ("data"=w1117:string)  [unwired: 1 in, 1 out]
        n150 = Number To Decimal String(number=w1096) -> (decimal integer string=w1114:string)  [unwired: 1 in]
        n151 = Number To Decimal String(number=w1095) -> (decimal integer string=w1131:string)  [unwired: 1 in]
        n152 = Number To Decimal String(number=w1094) -> (decimal integer string=w1130:string)  [unwired: 1 in]
        n153 = Number To Decimal String(number=w1091) -> (decimal integer string=w1124:string)  [unwired: 1 in]
        n154 = Number To Decimal String(number=w1093) -> (decimal integer string=w1120:string)  [unwired: 1 in]
        n155 = Number To Decimal String(number=w1092) -> (decimal integer string=w1121:string)  [unwired: 1 in]
        n156 = Number To Decimal String(number=w1090) -> (decimal integer string=w1125:string)  [unwired: 1 in]
        n157 = Subtract(x=w1097, y=w1096) -> (x-y=w1112:i32)
        n158 = Number To Decimal String(number=w1112) -> (decimal integer string=w1111:string)  [unwired: 1 in]
        n159 = Subtract(x=w1095, y=w1094) -> (x-y=w1119:i32)
        n160 = Subtract(x=w1093, y=w1092) -> (x-y=w1123:i32)
        n161 = Subtract(x=w1091, y=w1090) -> (x-y=w1127:i32)
        n162 = Number To Decimal String(number=w1119) -> (decimal integer string=w1118:string)  [unwired: 1 in]
        n163 = Number To Decimal String(number=w1123) -> (decimal integer string=w1122:string)  [unwired: 1 in]
        n164 = Number To Decimal String(number=w1127) -> (decimal integer string=w1126:string)  [unwired: 1 in]
        n165 = Build Array(w1117, w1113, w1116, w1115, w1114, w1111, w1131, w1130, w1118, w1120, w1121, w1122, w1124, w1125, w1126, w1128) -> (w1098:string[])
        "appended array 4" <- w1098
        n166 = Insert Into Array(array=w1134, new element=w1098) -> (w1135:string[][])  [unwired: 2 in]
      }
      n167 = call-poly <vilib>:"DB Tools Free Object.vi"("error in (no error)"=w1082, "recordset reference"=w1086) -> ("error out"=w1081:errorcluster, "connection reference"=w1085:T1)  [unwired: 8 in]
      n168 = call <vilib>:"DB Tools Close Connection.vi"("error in (no error)"=w1081, "connection reference"=w1085) -> ("error out"=→"error out 5":errorcluster)  [unwired: 5 in]
      n169 = Array Size(array=w1058) -> ()  [unwired: 1 out]
      n170 = Add Array Elements(numeric array=w1039) -> (sum=w1033:i32)
      n171 = Add Array Elements(numeric array=w1040) -> (sum=w1034:i32)
      n172 = Add Array Elements(numeric array=w1030) -> (sum=w1026:i32)
      n173 = Add Array Elements(numeric array=w1021) -> (sum=w1019:i32)
      n174 = Add Array Elements(numeric array=w1029) -> (sum=w1025:i32)
      n175 = Add Array Elements(numeric array=w1022) -> (sum=w1020:i32)
      n176 = Add Array Elements(numeric array=w1051) -> (sum=w1046:i32)
      n177 = Add Array Elements(numeric array=w1050) -> (sum=w1045:i32)
      n178 = Subtract(x=w1020, y=w1019) -> (x-y=w1018:i32)
      n179 = Subtract(x=w1026, y=w1025) -> (x-y=w1023:i32)
      n180 = Subtract(x=w1046, y=w1045) -> (x-y=w1038:i32)
      n181 = Subtract(x=w1034, y=w1033) -> (x-y=w1031:i32)
      n182 = Number To Decimal String(number=w1033) -> (decimal integer string=w1035:string)  [unwired: 1 in]
      n183 = Number To Decimal String(number=w1031) -> (decimal integer string=w1032:string)  [unwired: 1 in]
      n184 = Number To Decimal String(number=w1026) -> (decimal integer string=w1028:string)  [unwired: 1 in]
      n185 = Number To Decimal String(number=w1025) -> (decimal integer string=w1027:string)  [unwired: 1 in]
      n186 = Number To Decimal String(number=w1023) -> (decimal integer string=w1024:string)  [unwired: 1 in]
      n187 = Number To Decimal String(number=w1018) -> (decimal integer string=w1015:string)  [unwired: 1 in]
      n188 = Number To Decimal String(number=w1046) -> (decimal integer string=w1048:string)  [unwired: 1 in]
      n189 = Number To Decimal String(number=w1045) -> (decimal integer string=w1047:string)  [unwired: 1 in]
      n190 = Number To Decimal String(number=w1034) -> (decimal integer string=w1037:string)  [unwired: 1 in]
      n191 = Number To Decimal String(number=w1020) -> (decimal integer string=w1017:string)  [unwired: 1 in]
      n192 = Number To Decimal String(number=w1019) -> (decimal integer string=w1016:string)  [unwired: 1 in]
      n193 = Number To Decimal String(number=w1038) -> (decimal integer string=w1044:string)  [unwired: 1 in]
      n194 = Build Array(w1049, w1049, "Total :" ("element"), w1048, w1047, w1044, w1037, w1035, w1032, w1028, w1027, w1024, w1017, w1016, w1015, "") -> (w1043:string[])
      n195 = Insert Into Array(array=w1042, new element=w1043) -> (w1041:string[][])  [unwired: 2 in]
      n196 = local write "Table Control 3"(w1041) -> ()
    }
    frame #3 {
      w1542 = "macro1" ("macro name")
      w1577 = "MSTSummaryReport"
      w1543 = string[] ["Date", "Package", "Device", "Total", "Pass", "Fail", "Total", "Pass", "Fail", "Total", "Pass", "Fail", "Total", "Pass", "Fail", "Machine"] ("row headers")
      w1541 = cluster{"row":i32, "column":i32} {"row"=0, "column"=0} ("end (-1, -1)")
      w1590 = T3."Excel"  # Report Type
      # "Simulate UUT Testing"
      n197 = call <vilib>:"New Report.vi"("report type"=w1590, "template (empty)"="Report Template") -> ("report out"=w1586:refnum<class "NI_report.lvclass">, "error out"=w1585:errorcluster)  [unwired: 12 in]
      n198 = call <vilib>:"Excel Get Worksheet.vi"("report in"=w1586, "worksheet index (0)"=0, "error in (no error)"=w1585) -> ("report out"=w1536:refnum<class "NI_report.lvclass">, "error out"=w1535:errorcluster)  [unwired: 11 in]
      n199 = call <vilib>:"Excel Rename Worksheet.vi"("report in"=w1536, "worksheet name (\"\")"="LGE5331" ("worksheet name (\"\")"), "error in (no error)"=w1535) -> ("report out"=w1534:refnum<class "NI_report.lvclass">, "error out"=w1533:errorcluster)  [unwired: 11 in]
      n200 = Get Date/Time In Seconds() -> (seconds since 1Jan1904=w1522:timestamp)
      n201 = call-poly <vilib>:"Append Table to Report.vi"("report in"=w1534, "column headers"=w1543, "text data"="Table Control", "error in (no error)"=w1533) -> ("report out"=w1588:refnum<class "NI_report.lvclass">, "error out"=w1587:errorcluster)  [unwired: 8 in, 2 out]
      n202 = Get Date/Time String(seconds (now)=w1522) -> (date string=w1575:string, time string=w1529:string)  [unwired: 2 in]
      n203 = call <vilib>:"Excel Insert Cells.vi"("report in"=w1588, "error in (no error)"=w1587) -> ("report out"=w1584:refnum<class "NI_report.lvclass">, "error out"=w1583:errorcluster)  [unwired: 12 in]
      n204 = Concatenate Strings("Report Time :" ("string"), w1575, w1529) -> (w1526:string)
      n205 = call <vilib>:"Excel Easy Text.vi"("report in"=w1584, "text"=w1526, "start (-1, -1)"=w1541, "error in (no error)"=w1583) -> ("report out"=w1573:refnum<class "NI_report.lvclass">, "error out"=w1572:errorcluster)  [unwired: 7 in, 3 out]
      n206 = call <vilib>:"Excel Run Macro.vi"("report in"=w1573, "macro name"=w1542, "error in (no error)"=w1572) -> ("report out"=w1571:refnum<class "NI_report.lvclass">, "error out"=w1570:errorcluster)  [unwired: 10 in, 1 out]
      n207 = call <vilib>:"Excel Get Worksheet.vi"("report in"=w1571, "worksheet index (0)"=1, "error in (no error)"=w1570) -> ("report out"=w1568:refnum<class "NI_report.lvclass">, "error out"=w1567:errorcluster)  [unwired: 11 in]
      n208 = call-poly <vilib>:"Append Table to Report.vi"("report in"=w1568, "column headers"=w1543, "text data"="Table Control 2", "error in (no error)"=w1567) -> ("report out"=w1565:refnum<class "NI_report.lvclass">, "error out"=w1564:errorcluster)  [unwired: 8 in, 2 out]
      n209 = call <vilib>:"Excel Insert Cells.vi"("report in"=w1565, "error in (no error)"=w1564) -> ("report out"=w1563:refnum<class "NI_report.lvclass">, "error out"=w1562:errorcluster)  [unwired: 12 in]
      n210 = call <vilib>:"Excel Easy Text.vi"("report in"=w1563, "text"=w1526, "start (-1, -1)"=w1541, "error in (no error)"=w1562) -> ("report out"=w1561:refnum<class "NI_report.lvclass">, "error out"=w1560:errorcluster)  [unwired: 7 in, 3 out]
      n211 = call <vilib>:"Excel Run Macro.vi"("report in"=w1561, "macro name"=w1542, "error in (no error)"=w1560) -> ("report out"=w1559:refnum<class "NI_report.lvclass">, "error out"=w1558:errorcluster)  [unwired: 10 in, 1 out]
      n212 = call <vilib>:"Excel Rename Worksheet.vi"("report in"=w1559, "worksheet name (\"\")"="LGE5332" ("worksheet name (\"\")"), "error in (no error)"=w1558) -> ("report out"=w1545:refnum<class "NI_report.lvclass">, "error out"=w1544:errorcluster)  [unwired: 11 in]
      n213 = call <vilib>:"Excel Get Worksheet.vi"("report in"=w1545, "worksheet index (0)"=2, "error in (no error)"=w1544) -> ("report out"=w1556:refnum<class "NI_report.lvclass">, "error out"=w1555:errorcluster)  [unwired: 11 in]
      n214 = call-poly <vilib>:"Append Table to Report.vi"("report in"=w1556, "column headers"=w1543, "text data"="Table Control 3", "error in (no error)"=w1555) -> ("report out"=w1553:refnum<class "NI_report.lvclass">, "error out"=w1552:errorcluster)  [unwired: 8 in, 2 out]
      n215 = call <vilib>:"Excel Insert Cells.vi"("report in"=w1553, "error in (no error)"=w1552) -> ("report out"=w1551:refnum<class "NI_report.lvclass">, "error out"=w1550:errorcluster)  [unwired: 12 in]
      n216 = call <vilib>:"Excel Easy Text.vi"("report in"=w1551, "text"=w1526, "start (-1, -1)"=w1541, "error in (no error)"=w1550) -> ("report out"=w1549:refnum<class "NI_report.lvclass">, "error out"=w1548:errorcluster)  [unwired: 7 in, 3 out]
      n217 = call <vilib>:"Excel Run Macro.vi"("report in"=w1549, "macro name"=w1542, "error in (no error)"=w1548) -> ("report out"=w1547:refnum<class "NI_report.lvclass">, "error out"=w1546:errorcluster)  [unwired: 10 in, 1 out]
      n218 = call <vilib>:"Excel Rename Worksheet.vi"("report in"=w1547, "worksheet name (\"\")"="LGE5352" ("worksheet name (\"\")"), "error in (no error)"=w1546) -> ("report out"=w1524:refnum<class "NI_report.lvclass">, "error out"=w1523:errorcluster)  [unwired: 11 in]
      n219 = Format Date/Time String(time format string (%c)="%Y%m%d%H", seconds (now)=w1522) -> (date/time string=w1520:string)  [unwired: 1 in]
      n220 = Concatenate Strings(w1577, w1520, ".xls" ("string")) -> (w1578:string)
      n221 = Concatenate Strings(w1577, w1520) -> ()  [unwired: 1 out]
      n222 = call <vilib>:"Excel Get Worksheet.vi"("report in"=w1524, "worksheet index (0)"=0, "error in (no error)"=w1523) -> ("report out"=w1532:refnum<class "NI_report.lvclass">, "error out"=w1531:errorcluster)  [unwired: 11 in]
      n223 = Build Path(base path=path "o:/monitor/report", name or relative path=w1578) -> (appended path=w1576:path)
      n224 = call-dynamic "Save Report to File.vi"("report in"=w1532, "report file path"=w1576, "error in (no error)"=w1531) -> ("report out"=w1538:refnum<class "NI_report.lvclass">, "error out"=w1537:errorcluster)  [unwired: 11 in]
      n225 = call-dynamic "Dispose Report.vi"("report in"=w1538, "save changes? (F)"=FALSE, "error in (no error)"=w1537) -> ("error out"=→"error out 4":errorcluster)  [unwired: 12 in]
    }
    frame #4 {
      n226 = Index Array(array=w1594) -> (element=w1593:i32)  [unwired: 1 in]
      n227 = Greater?(x=w1593, y=1) -> (0:w1591:bool)
      n228 = case shown="True" w1591 {
        tunnel: w1596 -> [_ w1601]
        tunnel: w1595 -> [_ w1599]
        frame False {
        }
        frame True {
          (unwired) string[] ["yyliao@ptse.com.tw"] ("recipients")
          n229 = Concatenate Strings("******MStar Special  Monitor  Report from PTS*********" ("subject ([No Subject])"), w1599) -> (w1598:string)
          n230 = call <vilib>:"SMTP Email Send File.vi"("recipients"=string[] ["yyliao@ptse.com.tw", "E100@ptse.com.tw", "M110@ptse.com.tw", "whlee@ptse.com.tw", "color.yen@mstarsemi.com", "ch.yang@mstarsemi.com", "shang.liang@mstarsemi.com", "hy.chien@mstarsemi.com", "Allonsite@mstarsemi.com", "stanley.wang@mstarsemi.com", "zoe.huang@mstarsemi.com", "doris.lee@mstarsemi.com", "terry.lee@mstarsemi.com", "wj.hung@mstarsemi.com", "frank.liu@mstarsemi.com", "ywcheng@ptse.com.tw", "hzchen@ptse.com.tw", "jcwang@ptse.com.tw", "eric_fan@ptse.com.tw", "james@ptse.com.tw", "saulwang@ptse.com.tw", "jtwu@ptse.com.tw", "sam-cs.lin@mstarsemi.com", "hank.huang@mstarsemi.com", "peggylee@ptse.com.tw", "yi.lin@mstarsemi.com", "chialin.wang@mstarsemi.com "], "mail server"="192.168.1.17", "return address"="yyliao@ptse.com.tw", "subject ([No Subject])"=w1598, "message"="Dear sirs,\n\nAttached the Daily Report for your information,\n\nBest Regards,\n\n", "file path"=w1601, "binary? (F)"=TRUE, "MIME content-type (application/octet-stream)"="application/octet-stream") -> ()  [unwired: 6 in, 2 out]
        }
      }
    }
    frame #5 {
      n231 = Quit LabVIEW() -> ()  [unwired: 1 in]
    }
  }
